vi "configure.vi"(8 "error in (no error)":errorcluster, 11 "GenericPlugin in":refnum<class "StageFH090410SharedVariable.lvclass">) -> (0 "error out":errorcluster, 3 "GenericPlugin out":refnum<class "StageFH090410SharedVariable.lvclass">)   [LabVIEW 2010, in "StageFH090410SharedVariable.lvclass"]
doc: "The dynamic dispatch version of this VI loads and displays the configuration file associated with the plug-in object. The user modify and save the configuration data."
uses:
  StageFH090410SharedVariable.lvclass
  command_mode_enum.ctl
  StageFH090410SharedVariable.lvclass/StageFH090410SharedVariable.ctl
  common/classes/GenericComponent/GenericComponent/GenericComponent.lvclass
panel:
  in  "tolerance":dbl[unit]
  in  "command mode":T1
  in  "shared variable for move trigger":refnum<k21>="ni.var.psp://localhost/shared_variables/actual_position"
  in  "shared variable for position feedback":refnum<k21>="ni.var.psp://localhost/shared_variables/actual_position"
  in  "shared variable for motion command":refnum<k21>="ni.var.psp://localhost/shared_variables/actual_position"
  out "configuration":string
  in  "cancelButton":bool
  in  "okButton":bool
  # "Configure StageFH090410SharedVariable"
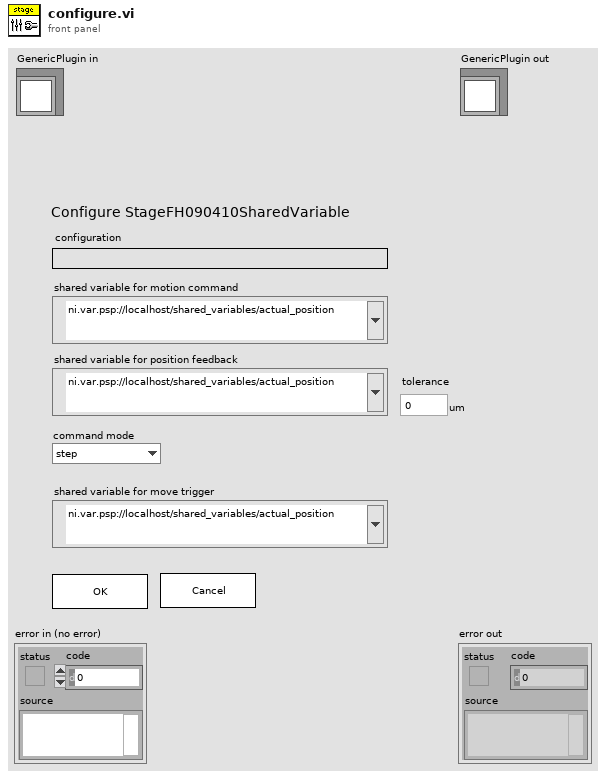
[diagram p1: front panel]
types:
  T1 = typedef "StageFH090410SharedVariable.lvclass/command_mode_enum.ctl" = enum16{"step", "absolute"}
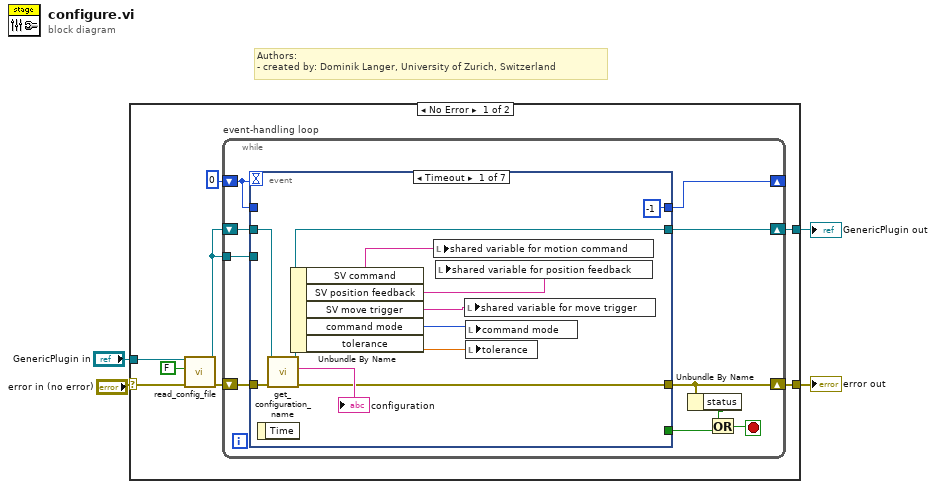
[diagram p0: block diagram]
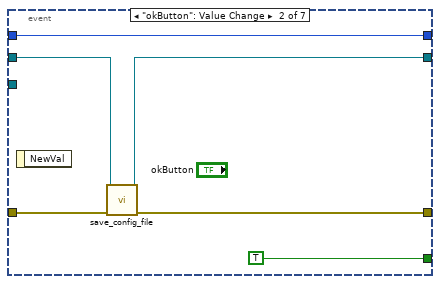
[diagram p2: hidden frame]
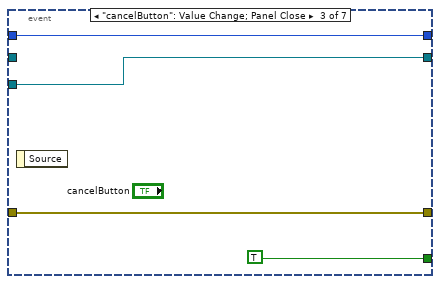
[diagram p3: hidden frame]
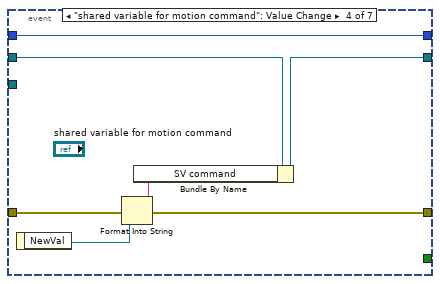
[diagram p4: hidden frame]
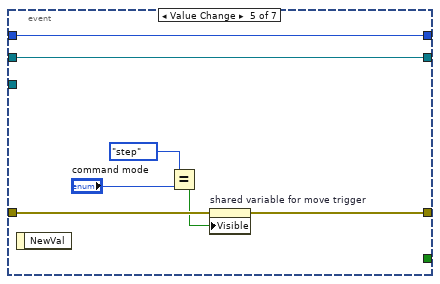
[diagram p5: hidden frame]
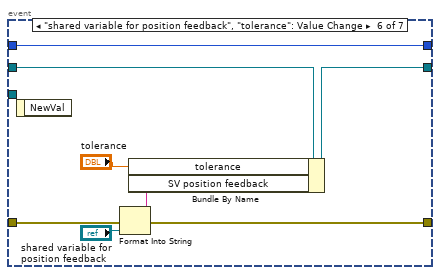
[diagram p6: hidden frame]
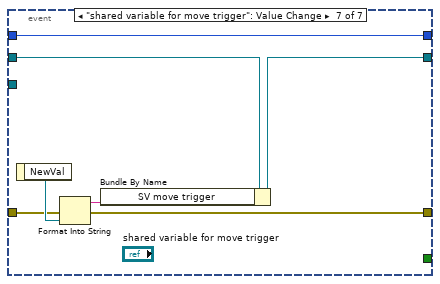
[diagram p7: hidden frame]
diagram:
  # "Authors: \n- created by: Dominik Langer, University of Zurich, Switzerland"
  n1 = case shown="No Error" "error in (no error)" {
    selector: "error in (no error)" -> [w10 w74]
    tunnel: "GenericPlugin in" -> [w8 w73]
    tunnel: [w12 w74] -> w2
    tunnel: [w11 w73] -> w1
    frame No Error {
      n2 = call-dynamic "read_config_file.vi"("error in (no error)"=w10, "force load?"=FALSE, "GenericPlugin in"=w8) -> ("error out"=w9:errorcluster, "GenericPlugin out"=w7:refnum<class "StageFH090410SharedVariable.lvclass">)  [unwired: 7 in]
      n3 = while "event-handling loop" {
        shift-right: [w19] -> w12
        shift-left: w9 -> [w20]
        shift-right: [w21] -> w11
        shift-left: w7 -> [w22]
        tunnel: w7 -> [w15]
        shift-right: [w13] -> _
        shift-left: 0 -> [w14]
        stop <- w16 stop-if-true
        n4 = event shown="[0] Timeout" {
          selector: _ -> [_ _ _ _ _ _ _]
          dyn-events: _ -> [_ _ _ _ _ _ _]
          timeout: w14 -> [_ _ _ _ _ _ _]
          tunnel: w22 -> [w32 w35 _ w50 w57 w62 w67]
          tunnel: [w30 w34 w42 w49 w57 w61 w66] -> w21
          tunnel: [w29 w36 w43 w47 w54 w63 w69] -> w19
          tunnel: w20 -> [w33 w37 w43 w48 w55 w64 w70]
          tunnel: [_ TRUE TRUE _ _ _ _] -> w17
          tunnel: w15 -> [_ _ w42 _ _ _ _]
          tunnel: w14 -> [_ w38 w40 w44 w56 w60 w72]
          tunnel: [-1 w38 w40 w44 w56 w60 w72] -> w13
          event Timeout {
            n5 = event-data() -> ()  [unwired: 1 in, 1 out]
            n6 = call "get_configuration_name.vi"("error in (no error)"=w33, "GenericPlugin.lvclass in"=w32) -> ("error out"=w29:errorcluster, "configuration name"=→"configuration":string, "GenericPlugin.lvclass out"=w30:refnum<class "StageFH090410SharedVariable.lvclass">)  [unwired: 7 in]
            n7 = Unbundle By Name(w30) -> ("SV command"=w26:string, "SV position feedback"=w27:string, "SV move trigger"=w25:string, "command mode"=w24:T1, "tolerance"=w23:dbl[unit])
            n8 = local write "shared variable for motion command"(w26) -> ()
            n9 = local write "shared variable for position feedback"(w27) -> ()
            n10 = local write "shared variable for move trigger"(w25) -> ()
            n11 = local write "command mode"(w24) -> ()
            n12 = local write "tolerance"(w23) -> ()
          }
          event "okButton": Value Change {
            n13 = event-data() -> ()  [unwired: 1 in, 1 out]
            n14 = call-dynamic "save_config_file.vi"("error in (no error)"=w37, "GenericPlugin in"=w35) -> ("error out"=w36:errorcluster, "GenericPlugin out"=w34:refnum<class "StageFH090410SharedVariable.lvclass">)  [unwired: 8 in]
          }
          event "cancelButton": Value Change; Panel Close {
            n15 = event-data() -> ()  [unwired: 1 in, 1 out]
          }
          event "shared variable for motion command": Value Change {
            n16 = event-data() -> ("NewVal"=w45:refnum<k21>)  [unwired: 1 in]
            n17 = Format Into String(error in=w48, w45) -> (resulting string=w46:string, error out=w47:errorcluster)  [unwired: 2 in]
            n18 = Bundle By Name(cluster=w50, "SV command"=w46) -> (w49:refnum<class "StageFH090410SharedVariable.lvclass">)
          }
          event Value Change {
            n19 = event-data() -> ()  [unwired: 1 in, 1 out]
            n20 = Equal?(x=command_mode_enum."step", y="command mode") -> (x = y?=w51:bool)
            n21 = property on="shared variable for move trigger" class="Variable (strict)"(error in=w55, "Visible"=w51) -> (error out=w54:errorcluster)  [unwired: 1 in, 1 out]
          }
          event "shared variable for position feedback", "tolerance": Value Change {
            n22 = event-data() -> ()  [unwired: 1 in, 1 out]
            n23 = Format Into String(error in=w64, "shared variable for position feedback") -> (resulting string=w65:string, error out=w63:errorcluster)  [unwired: 2 in]
            n24 = Bundle By Name(cluster=w62, "tolerance"="tolerance", "SV position feedback"=w65) -> (w61:refnum<class "StageFH090410SharedVariable.lvclass">)
          }
          event "shared variable for move trigger": Value Change {
            n25 = event-data() -> ("NewVal"=w71:refnum<k21>)  [unwired: 1 in]
            n26 = Format Into String(error in=w70, w71) -> (resulting string=w68:string, error out=w69:errorcluster)  [unwired: 2 in]
            n27 = Bundle By Name(cluster=w67, "SV move trigger"=w68) -> (w66:refnum<class "StageFH090410SharedVariable.lvclass">)
          }
        }
        n28 = Unbundle By Name(w19) -> ("status"=w18:bool)
        n29 = Or(x=w18, y=w17) -> (x .or. y?=w16:bool)
      }
    }
    frame Error {
    }
  }
  "error out" <- w2
  "GenericPlugin out" <- w1
